vi "receiver_udp.vi"() -> ()   [LabVIEW 2022 SP3]
panel:
  out "binary num":string
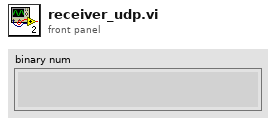
[diagram p1: front panel]
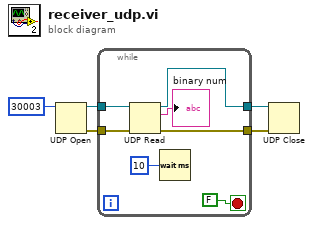
[diagram p0: block diagram]
diagram:
  n1 = UDP Open(11:u16 30003 ("port")) -> (port=w4:refnum<k16>, 0:w3:errorcluster)  [unwired: 4 in, 1 out]
  n2 = while {
    tunnel: w4 -> [w12]
    tunnel: w3 -> [w11]
    tunnel: [w8] -> w2
    tunnel: [w7] -> w1
    stop <- FALSE stop-if-true
    n3 = UDP Read(connection ID=w12, 8:w11) -> (data out=→"binary num":string, error out=w7:errorcluster, 3:w8:refnum<k16>)  [unwired: 2 in, 2 out]
    n4 = Wait (ms)(milliseconds to wait=u32 10) -> ()  [unwired: 1 out]
  }
  n5 = UDP Close(connection ID=w2, 8:w1) -> ()  [unwired: 2 out]
